vi "write Array of Doubles.vi"(9 "values":cluster{"Array":dbl[]}[](array[cluster]), 10 "indices":i32[](array[numeric]), 11 "data table in":T1) -> (3 "data table out":T1)   [LabVIEW 2013, in "data bus values.lvlib"]
doc: "Writes a set of values to the data table. Requires an index for every value."
uses:
  data bus values.lvlib
  data table.ctl
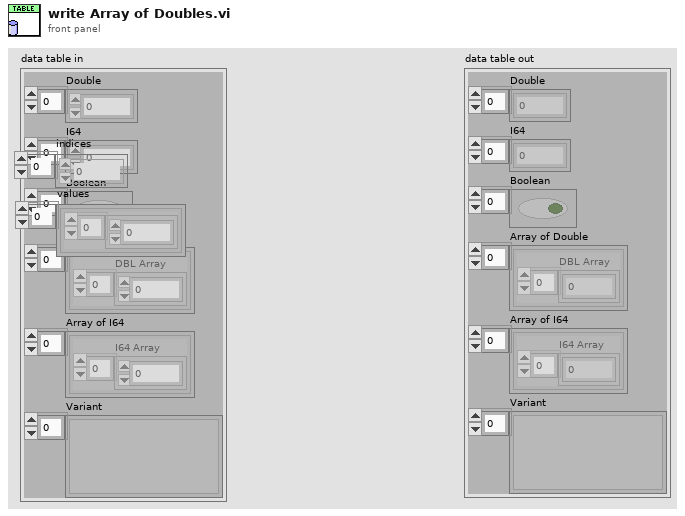
[diagram p1: front panel]
types:
  T1 = typedef "data bus values.lvlib/data table.ctl" = cluster{"Double":dbl[], "I64":i64[], "Boolean":bool[], "Array of Double":cluster{"DBL Array":dbl[]}[], "Array of I64":cluster{"I64 Array":i64[]}[], "Variant":variant[]}
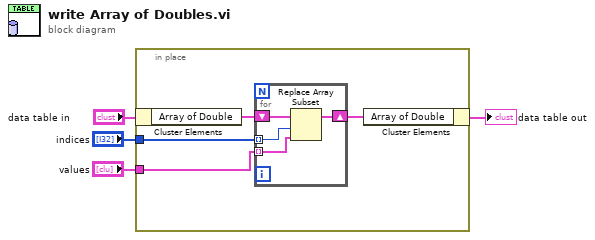
[diagram p0: block diagram]
diagram:
  n1 = in-place {
    in-place-border: "indices" -> [w6]
    in-place-border: "values" -> [w5]
    n2 = in-place-cluster #1("data table in") -> ("Array of Double"=w8:cluster{"DBL Array":dbl[]}[])
    n3 = for {
      tunnel: w6 -> [w12] mode=indexing
      tunnel: w5 -> [w11] mode=indexing
      shift-right: [w9] -> w7
      shift-left: w8 -> [w10]
      n4 = Replace Array Subset(array=w10, new element=w11, index=w12) -> (w9:cluster{"DBL Array":dbl[]}[])
    }
    n5 = in-place-cluster #1("Array of Double"=w7) -> (→"data table out":T1)
  }
